vi "Get Scene Object Refnum.vi"(8 "error in (no error)":errorcluster, 11 "XRay Beam in":refnum<class "XRay Beam.lvclass">) -> (0 "error out":errorcluster, 2 "Beam":refnum<vi>, 3 "XRay Beam out":refnum<class "XRay Beam.lvclass">)   [LabVIEW 2026, in "XRay Beam.lvclass"]
uses:
  XRay Beam.lvclass
  XRay Beam.lvclass/XRay Beam.ctl
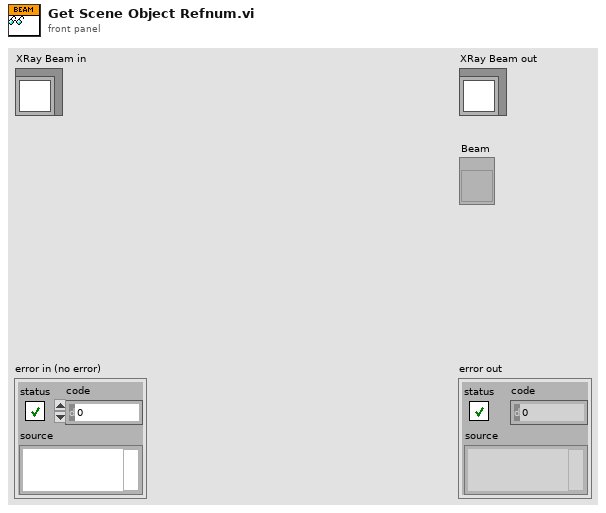
[diagram p1: front panel]
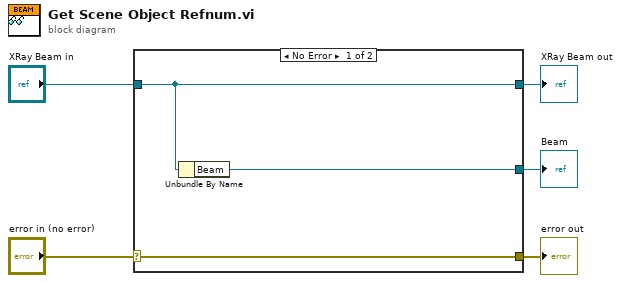
[diagram p0: block diagram]
diagram:
  n1 = case shown="No Error" "error in (no error)" {
    selector: "error in (no error)" -> [w8 w9]
    tunnel: [w8 w9] -> w4
    tunnel: [w7 w10] -> w2
    tunnel: "XRay Beam in" -> [w7 w10]
    tunnel: [w6 _] -> w1
    frame No Error {
      n2 = Unbundle By Name(w7) -> ("Beam"=w6:refnum<vi>)
    }
    frame Error {
    }
  }
  "error out" <- w4
  "XRay Beam out" <- w2
  "Beam" <- w1
